vi "button elapsed time.vi"(11 "Button":bool) -> (2 "Elapsed time":dbl)   [LabVIEW 2011]
panel:
  out "Start Time":timestamp
  in  "Last Botton":bool
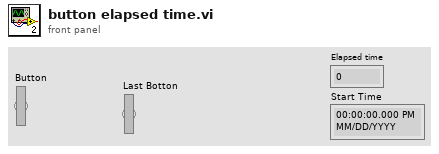
[diagram p1: front panel]
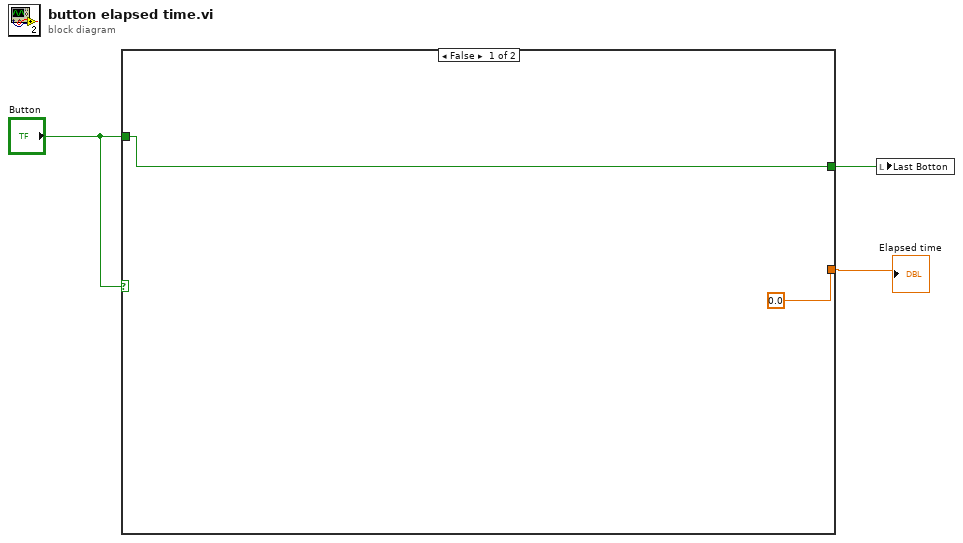
[diagram p0: block diagram]
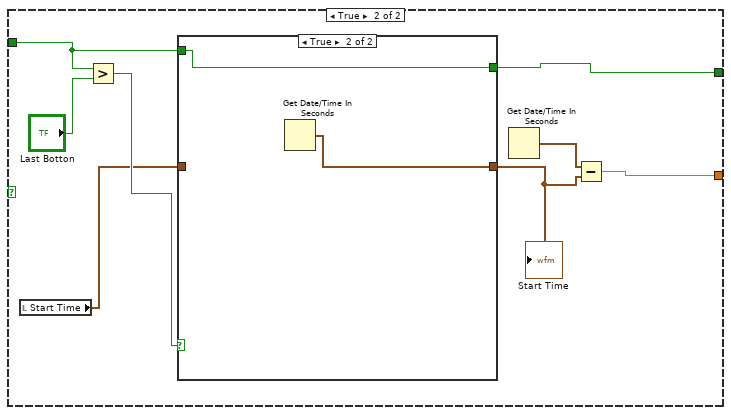
[diagram p2: hidden frame]
diagram:
  n1 = case shown="False" "Button" {
    tunnel: "Button" -> [w4 w10]
    tunnel: [0.0 ("Elapsed time") w7] -> w2
    tunnel: [w4 w6] -> w1
    frame False {
    }
    frame True {
      n2 = local read "Start Time"() -> (w11:timestamp)
      n3 = Greater?(x=w10, y="Last Botton") -> (0:w12:bool)
      n4 = case shown="True" w12 {
        tunnel: [w15 w17] -> w9
        tunnel: w11 -> [w15 _]
        tunnel: w10 -> [w14 w16]
        tunnel: [w14 w16] -> w6
        frame False {
        }
        frame True {
          n5 = Get Date/Time In Seconds() -> (seconds since 1Jan1904=w17:timestamp)
        }
      }
      "Start Time" <- w9
      n6 = Get Date/Time In Seconds() -> (seconds since 1Jan1904=w8:timestamp)
      n7 = Subtract(x=w8, y=w9) -> (x-y=w7:dbl)
    }
  }
  "Elapsed time" <- w2
  n8 = local write "Last Botton"(w1) -> ()
